vi "Create_directory_path.vi"(2 "error in (no error)":errorcluster, 3 "Path name":path) -> (0 "error out":errorcluster, 1 "Path name Out":path)   [LabVIEW 2011]
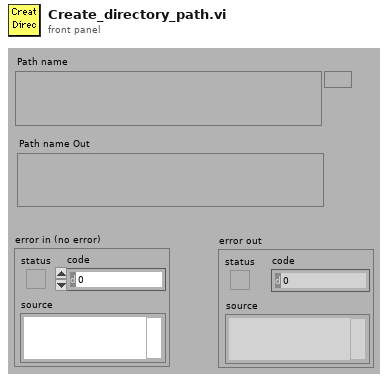
[diagram p1: front panel]
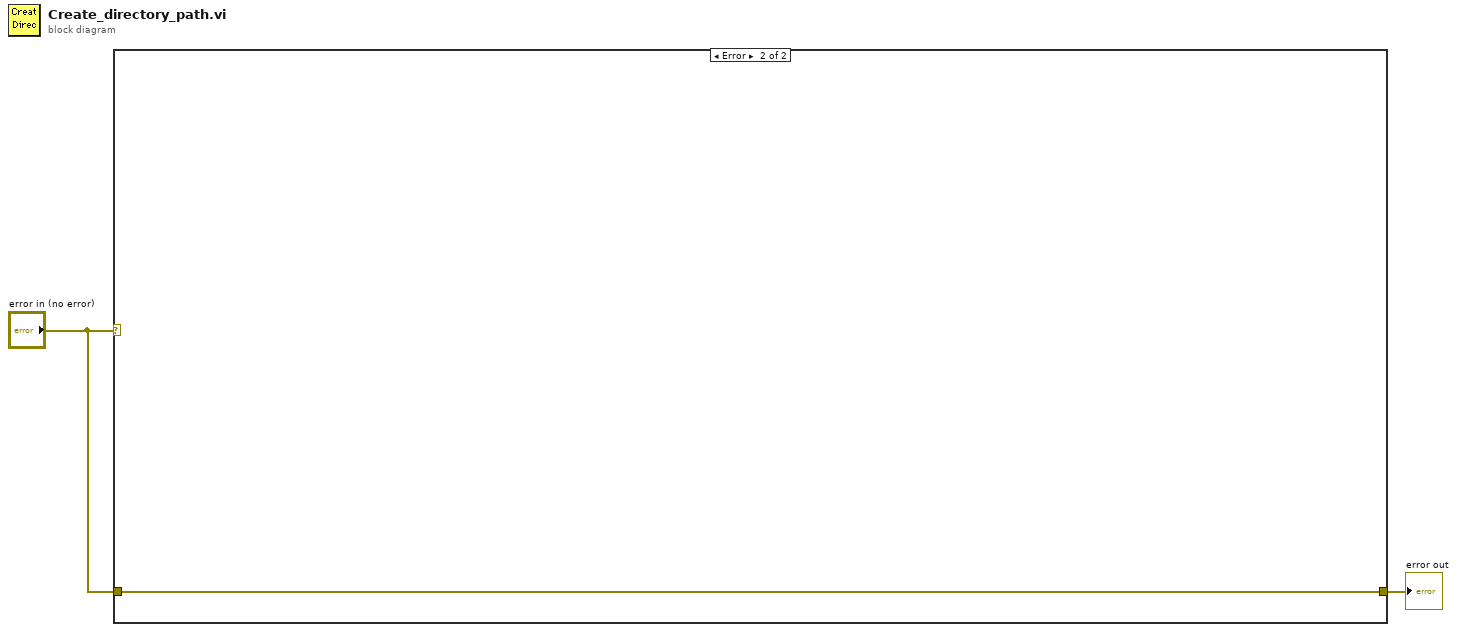
[diagram p0: block diagram]
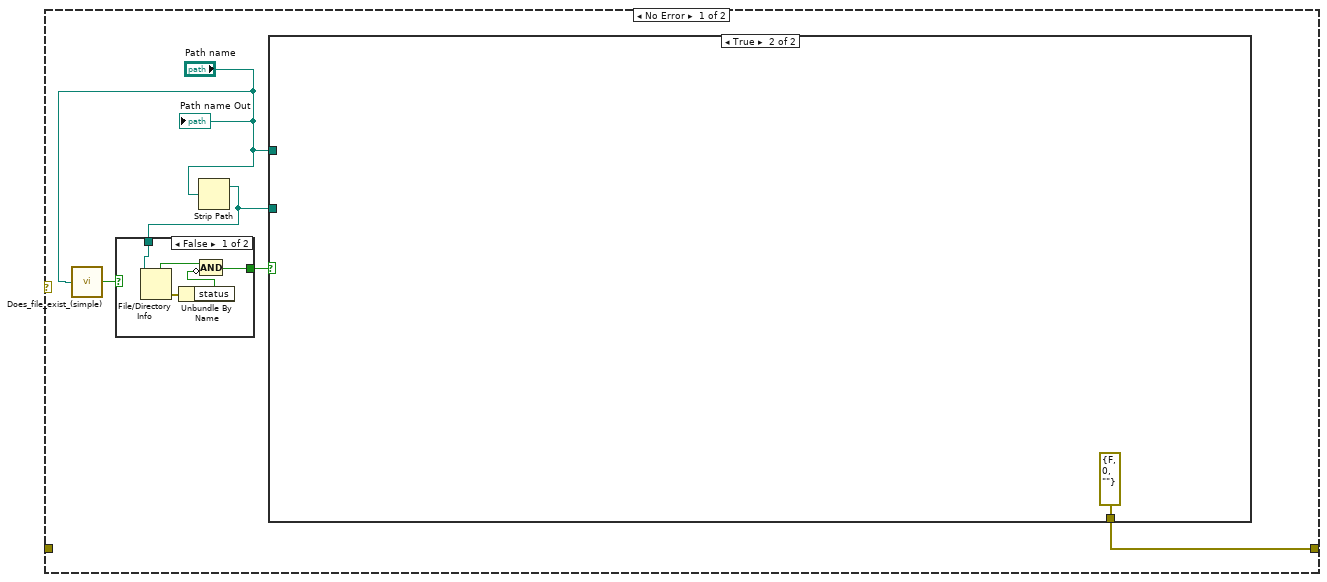
[diagram p2: hidden frame]
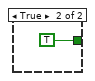
[diagram p3: hidden frame]
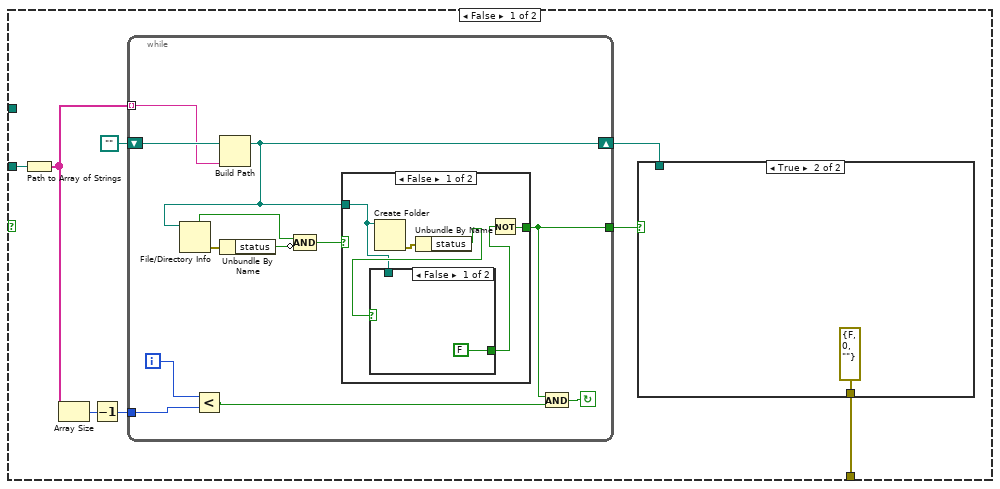
[diagram p4: hidden frame]
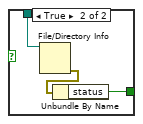
[diagram p5: hidden frame]
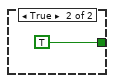
[diagram p6: hidden frame]
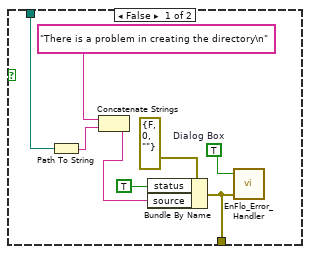
[diagram p7: hidden frame]
diagram:
  n1 = case shown="Error" "error in (no error)" {
    tunnel: [w3 w54] -> w2
    tunnel: "error in (no error)" -> [_ w54]
    frame No Error {
      n2 = call "Does_file_exist_(simple).vi"("Pathname"="Path name") -> ("exists?"=w5:bool)
      n3 = Strip Path(path="Path name") -> (stripped path=w6:path)  [unwired: 1 out]
      n4 = case shown="False" w5 {
        tunnel: [w11 TRUE] -> w7
        tunnel: w6 -> [w8 _]
        frame False {
          n5 = File/Directory Info(path=w8) -> (directory=w9:bool, error out=w12:errorcluster)  [unwired: 1 in, 5 out]
          n6 = Unbundle By Name(w12) -> ("status"=w10:bool)
          n7 = Compound Arithmetic op=AND(w9, invert w10) -> (w11:bool)
        }
        frame True {
        }
      }
      n8 = case shown="True" w7 {
        tunnel: "Path name" -> [_ _]
        tunnel: w6 -> [w16 _]
        tunnel: [w14 errorcluster {"status"=FALSE, "code"=0, "source"=""} ("error in (no error)")] -> w3
        frame False {
          n9 = Path to Array of Strings(0:w16) -> (2:w20:string[])  [unwired: 1 out]
          n10 = Array Size(array=w20) -> (size(s)=w15:i32)
          n11 = Decrement(x=w15) -> (x-1=w17:i32)
          n12 = while {
            tunnel: [w27] -> w19
            tunnel: w17 -> [w30]
            shift-left: path "" ("appended path") -> [w33]
            shift-right: [w26] -> w18
            tunnel: w20 -> [w32] mode=indexing
            i -> [w31]
            stop <- w28 continue-if-true
            n13 = Less?(x=w31, y=w30) -> (x < y?=w29:bool)
            n14 = Build Path(base path=w33, name or relative path=w32) -> (appended path=w26:path)
            n15 = File/Directory Info(path=w26) -> (directory=w23:bool, error out=w25:errorcluster)  [unwired: 1 in, 5 out]
            n16 = Unbundle By Name(w25) -> ("status"=w24:bool)
            n17 = Compound Arithmetic op=AND(w23, invert w24) -> (w22:bool)
            n18 = case shown="False" w22 {
              tunnel: w26 -> [w35 _]
              tunnel: [w37 TRUE] -> w27
              frame False {
                n19 = Create Folder(path (use dialog)=w35) -> (error out=w38:errorcluster)  [unwired: 1 in, 3 out]
                n20 = Unbundle By Name(w38) -> ("status"=w36:bool)
                n21 = case shown="False" w36 {
                  tunnel: w35 -> [_ w42]
                  tunnel: [FALSE ("status") w40] -> w34
                  frame False {
                  }
                  frame True {
                    n22 = File/Directory Info(path=w42) -> (error out=w41:errorcluster)  [unwired: 1 in, 6 out]
                    n23 = Unbundle By Name(w41) -> ("status"=w40:bool)
                  }
                }
                n24 = Not(x=w34) -> (.not. x?=w37:bool)
              }
              frame True {
              }
            }
            n25 = And(x=w27, y=w29) -> (x .and. y?=w28:bool)
          }
          n26 = case shown="True" w19 {
            tunnel: w18 -> [w51 _]
            tunnel: [w44 errorcluster {"status"=FALSE, "code"=0, "source"=""} ("error in (no error)")] -> w14
            frame False {
              w47 = TRUE  # Dialog Box
              n27 = Path To String(path=w51) -> (string=w49:string)
              n28 = Concatenate Strings("There is a problem in creating the directory\n", w49) -> (w45:string)
              n29 = Bundle By Name(cluster=errorcluster {"status"=FALSE, "code"=0, "source"=""} ("error in (no error)"), "status"=TRUE ("Bundle Element"), "source"=w45) -> (w44:errorcluster)
              n30 = call "EnFlo_Error_Handler.vi"("error in (no error)"=w44, "Dialog Box (T)"=w47) -> ()  [unwired: 1 in, 3 out]
            }
            frame True {
            }
          }
        }
        frame True {
        }
      }
      "Path name Out" <- "Path name"
    }
    frame Error {
    }
  }
  "error out" <- w2
